vi "Log Result.vi"(8 "error in (no error)":errorcluster, 10 "tdms file":refnum<k34>, 11 "Mag Lab Result in":refnum<class "Mag Lab Result.lvclass">) -> (0 "error out":errorcluster, 2 "tdms file out":refnum<k34>, 3 "Mag Lab Result out":refnum<class "Mag Lab Result.lvclass">)   [LabVIEW 2015, in "Mag Lab Result.lvclass"]
uses:
  Mag Lab Result.lvclass
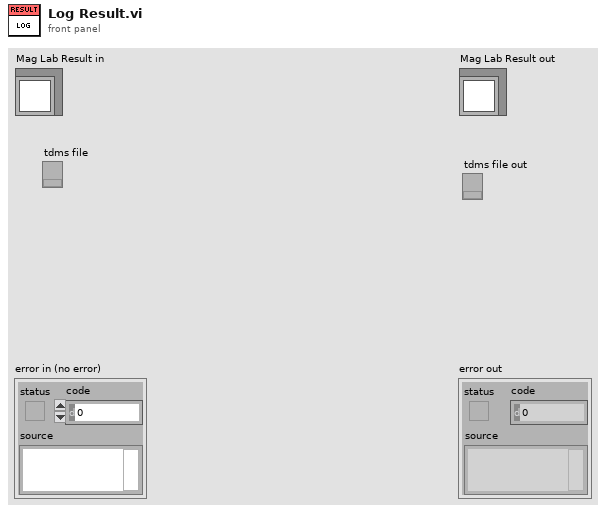
[diagram p1: front panel]
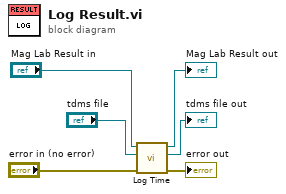
[diagram p0: block diagram]
diagram:
  n1 = call-dynamic "Log Time.vi"("error in (no error)"="error in (no error)", "tdms file"="tdms file", "Mag Lab Result in"="Mag Lab Result in") -> ("error out"=→"error out":errorcluster, "tdms file out"=→"tdms file out":refnum<k34>, "Mag Lab Result out"=→"Mag Lab Result out":refnum<class "Mag Lab Result.lvclass">)  [unwired: 6 in]
